vi "Create Frame Point Array.vi"(9 "Height (m)":dbl, 10 "Width (m)":dbl, 11 "Origin Point":T1 {"Latitude" format="%#_10g"; "Longitude" format="%#_10g"}) -> (3 "Frame Points":T1[](array[typedef]) {"Latitude" format="%#_10g"; "Longitude" format="%#_10g"})   [LabVIEW 2014]
uses:
  Lat Long Conversion/Controls/PointLatLon.ctl
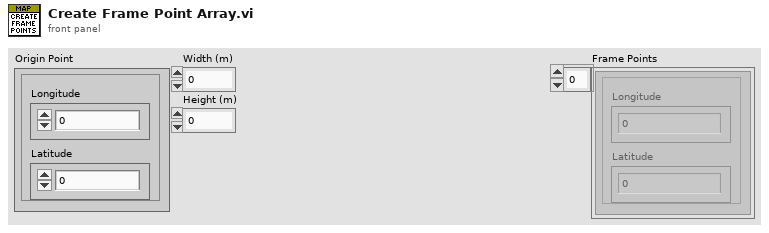
[diagram p1: front panel]
types:
  T1 = typedef "PointLatLon.ctl" = cluster{"Longitude":dbl, "Latitude":dbl}
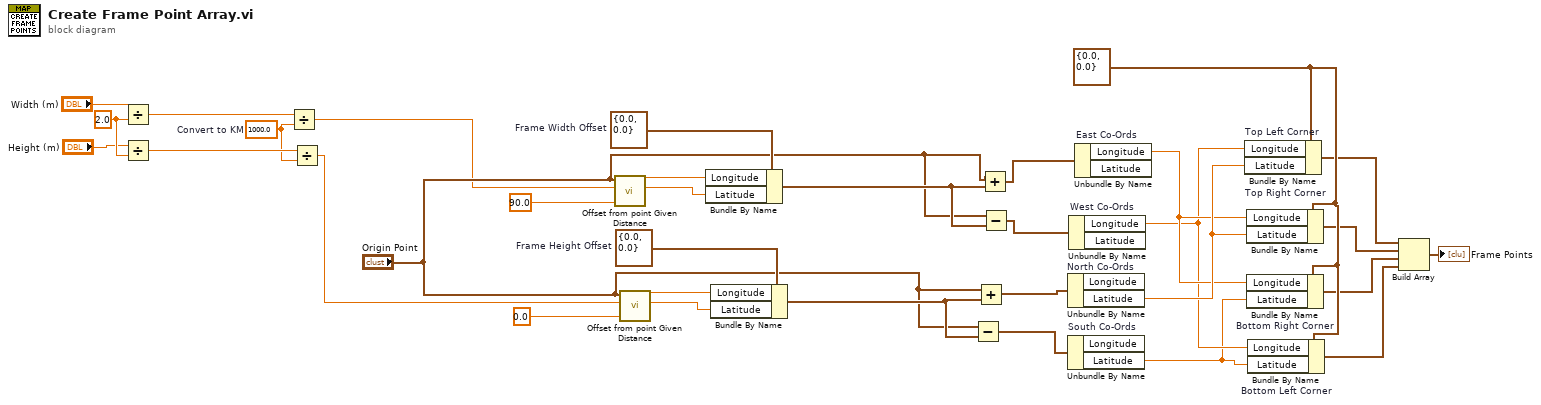
[diagram p0: block diagram]
diagram:
  w6 = 1000.0  # Convert to KM
  w9 = 2.0 ("y")
  w22 = T1 {"Longitude"=0.0, "Latitude"=0.0}  # Frame Width Offset
  w28 = T1 {"Longitude"=0.0, "Latitude"=0.0}  # Frame Height Offset
  w33 = T1 {"Longitude"=0.0, "Latitude"=0.0} ("Origin Point")
  n1 = Divide(x="Width (m)", y=w9) -> (x/y=w8:dbl)
  n2 = Divide(x="Height (m)", y=w9) -> (x/y=w7:dbl)
  n3 = Divide(x=w8, y=w6) -> (x/y=w5:dbl)
  n4 = Divide(x=w7, y=w6) -> (x/y=w4:dbl)
  n5 = call "Offset from point Given Distance.vi"("Bearing (clockwise from North)"=90.0, "Distance (km)"=w5, "Origin Point"="Origin Point") -> ("Lat Offset"=w24:dbl, "Lon Offset"=w23:dbl)  [unwired: 7 in]
  n6 = call "Offset from point Given Distance.vi"("Bearing (clockwise from North)"=0.0, "Distance (km)"=w4, "Origin Point"="Origin Point") -> ("Lat Offset"=w26:dbl, "Lon Offset"=w27:dbl)  [unwired: 7 in]
  n7 = Bundle By Name(cluster=w22, "Longitude"=w23, "Latitude"=w24) -> (w20:T1)
  n8 = Bundle By Name(cluster=w28, "Longitude"=w27, "Latitude"=w26) -> (w19:T1)
  n9 = Subtract(x="Origin Point", y=w19) -> (x-y=w17:T1)
  n10 = Add(x="Origin Point", y=w19) -> (x+y=w18:T1)
  n11 = Add(x="Origin Point", y=w20) -> (x+y=w15:T1)
  n12 = Subtract(x="Origin Point", y=w20) -> (x-y=w16:T1)
  n13 = Unbundle By Name "North Co-Ords"(w18) -> ("Latitude"=w14:dbl)  [unwired: 1 out]
  n14 = Unbundle By Name "South Co-Ords"(w17) -> ("Latitude"=w11:dbl)  [unwired: 1 out]
  n15 = Unbundle By Name "West Co-Ords"(w16) -> ("Longitude"=w12:dbl)  [unwired: 1 out]
  n16 = Unbundle By Name "East Co-Ords"(w15) -> ("Longitude"=w13:dbl)  [unwired: 1 out]
  n17 = Bundle By Name "Top Left Corner"(cluster=w33, "Longitude"=w12, "Latitude"=w14) -> (w32:T1)
  n18 = Bundle By Name "Top Right Corner"(cluster=w33, "Longitude"=w13, "Latitude"=w14) -> (w31:T1)
  n19 = Bundle By Name "Bottom Right Corner"(cluster=w33, "Longitude"=w13, "Latitude"=w11) -> (w30:T1)
  n20 = Bundle By Name "Bottom Left Corner"(cluster=w33, "Longitude"=w12, "Latitude"=w11) -> (w29:T1)
  n21 = Build Array(w32, w31, w30, w29) -> (→"Frame Points":T1[])
